vi "Handle Notification.vi"(8 "error in (no error)":errorcluster, 9 "Payload":string, 10 "Notification Type":string, 11 "CycleCounter in":refnum<class "RPM Measurement.lvclass">) -> (0 "error out":errorcluster, 3 "CycleCounter out":refnum<class "RPM Measurement.lvclass">)   [LabVIEW 2020, in "RPM Measurement.lvlib" / "RPM Measurement.lvclass"]
uses:
  RPM Measurement.lvclass
  RPM Measurement.lvclass/RPM Measurement.ctl
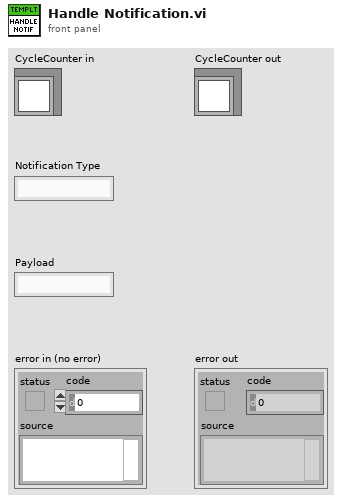
[diagram p1: front panel]
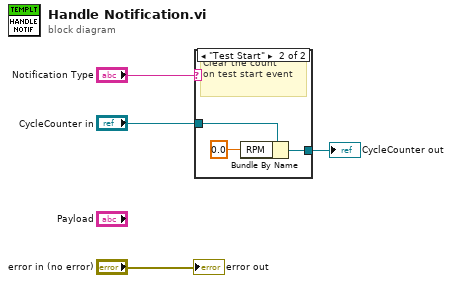
[diagram p0: block diagram]
diagram:
  n1 = case shown="\"Test Start\"" "Notification Type" {
    tunnel: "CycleCounter in" -> [w5 w8]
    tunnel: [w5 w6] -> w2
    frame Default {
    }
    frame "Test Start" {
      # "Clear the count\non test start event"
      n2 = Bundle By Name(cluster=w8, "RPM"=0.0 ("Count")) -> (w6:refnum<class "RPM Measurement.lvclass">)
    }
  }
  "CycleCounter out" <- w2
  "error out" <- "error in (no error)"
